vi "WPI_RobotDriveDelayAndUpdateSafety_2168.vi"(6 "Feed time (s)":dbl, 10 "Delay (s)":dbl, 11 "RobotDriveDevRef":string) -> (3 "RobotDriveDevRef":string)   [LabVIEW 2017]
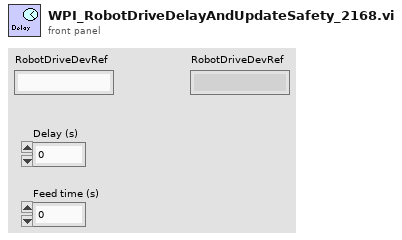
[diagram p1: front panel]
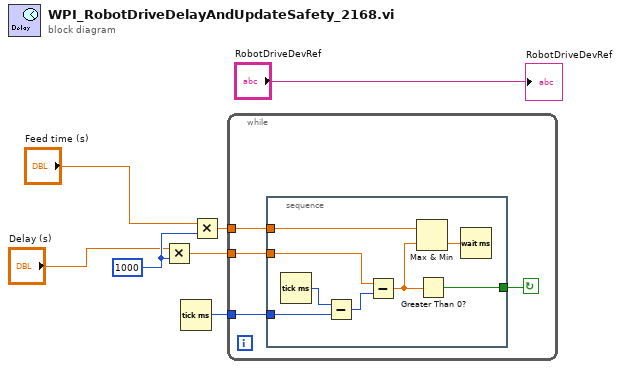
[diagram p0: block diagram]
diagram:
  w4 = 1000
  n1 = Multiply(x="Delay (s)", y=w4) -> (x*y=w5:dbl)
  n2 = Tick Count (ms)() -> (millisecond timer value=w7:u32)
  n3 = Multiply(x="Feed time (s)", y=w4) -> (x*y=w6:dbl)
  n4 = while {
    tunnel: w5 -> [w9]
    tunnel: w6 -> [w10]
    tunnel: w7 -> [w11]
    stop <- w8 continue-if-true
    n5 = stacked-sequence {
      tunnel: w11 -> [w19]
      tunnel: w10 -> [w18]
      tunnel: w9 -> [w16]
      tunnel: [w12] -> w8
      frame #0 {
        n6 = Tick Count (ms)() -> (millisecond timer value=w14:u32)
        n7 = Subtract(x=w14, y=w19) -> (x-y=w15:u32)
        n8 = Subtract(x=w16, y=w15) -> (x-y=w13:dbl)
        n9 = Max & Min(x=w18, y=w13) -> (min(x,y)=w17:dbl)  [unwired: 1 out]
        n10 = Greater Than 0?(x=w13) -> (x > 0?=w12:bool)
        n11 = Wait (ms)(milliseconds to wait=w17) -> ()  [unwired: 1 out]
      }
    }
  }
  "RobotDriveDevRef" <- "RobotDriveDevRef"
